vi "zad1.vi"() -> ()   [LabVIEW 2018]
uses:
  <vilib>/sound2/lvsound2.llb/Sampling Mode.ctl
  <vilib>/sound2/lvsound2.llb/Sound Data Format.ctl
  <vilib>/sound2/lvsound2.llb/Sound Output Set Volume (Single).vi
  <vilib>/sound2/lvsound2.llb/Sound Output Write (DBL Single).vi
  <vilib>/sound2/lvsound2.llb/Sound Input Read (DBL).vi
  <vilib>/measure/NI_MABase.lvlib
panel:
  in  "Stop":bool
  out "Waveform Graph 2":waveform(dbl)[](graph)
  out "Waveform Graph":waveform(dbl)(graph)
  in  "frequency":dbl(slide)=10.0 scale=200.0..2000.0
  in  "volume":dbl(knob)=100.0 scale=0.0..100.0
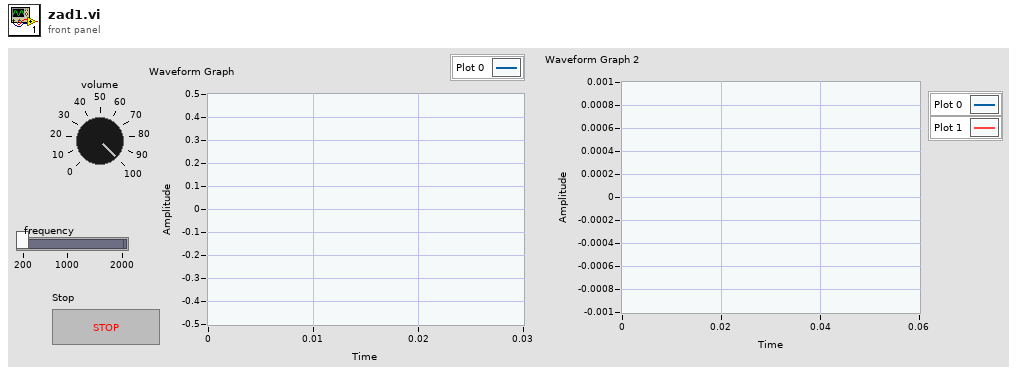
[diagram p1: front panel]
types:
  T1 = typedef "Sound Data Format.ctl" = cluster{"sample rate (S/s)":dbl, "number of channels":i32, "bits per sample":i32}
  T2 = typedef "Sampling Mode.ctl" = i32
  T3 = typedef "Sound Output Task ID.ctl" = u32
  T4 = typedef "Sound Input Task ID.ctl" = u32
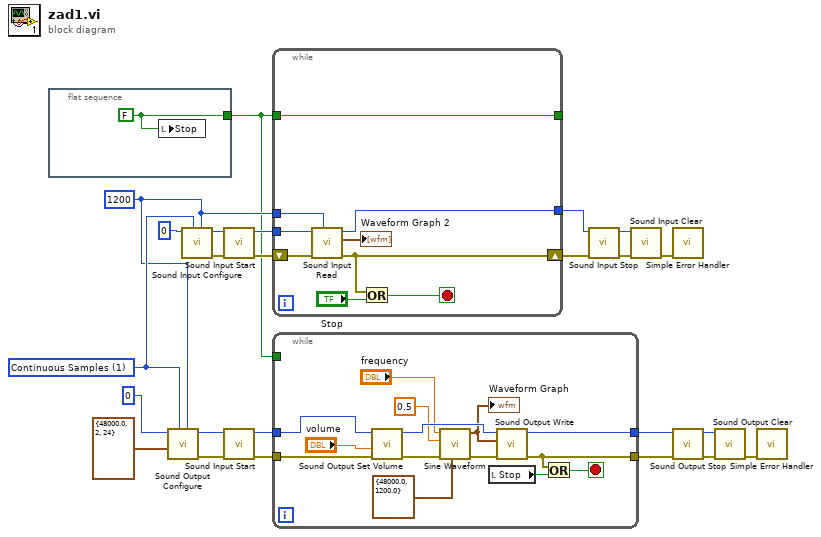
[diagram p0: block diagram]
diagram:
  w11 = 1200 ("number of samples/ch")
  w15 = T2 1 items=["Finite Samples", "Continuous Samples"] ("sample mode")
  n1 = flat-sequence {
    tunnel: [w25] -> w3
    frame #0 {
      w25 = FALSE
      n2 = local write "Stop"(w25) -> ()
    }
  }
  n3 = call <vilib>:"Sound Output Configure.vi"("number of samples/ch"=w11, "sample mode"=w15, "sound format"=T1 {"sample rate (S/s)"=48000.0, "number of channels"=2, "bits per sample"=24}, "device ID"=u32 0) -> ("error out"=w5:errorcluster, "task ID"=w6:T3)  [unwired: 6 in]
  n4 = call <vilib>:"Sound Input Configure.vi"("number of samples/ch"=w11, "sample mode"=w15, "device ID"=u32 0) -> ("error out"=w18:errorcluster, "task ID"=w19:T4)  [unwired: 7 in]
  n5 = call <vilib>:"Sound Input Start.vi"("error in (no error)"=w18, "task ID"=w19) -> ("error out"=w16:errorcluster, "task ID out"=w17:T4)  [unwired: 8 in]
  n6 = call <vilib>:"Sound Input Start.vi"("error in (no error)"=w5, "task ID"=w6) -> ("error out"=w7:errorcluster, "task ID out"=w8:T4)  [unwired: 8 in]
  n7 = while {
    tunnel: w17 -> [w34]
    tunnel: w11 -> [w31]
    shift-right: [w29] -> w10
    shift-left: w16 -> [w33]
    tunnel: [w27] -> w4
    tunnel: [w26] -> _
    tunnel: w3 -> [w26]
    stop <- w28 stop-if-true
    n8 = call-poly <vilib>:"Sound Input Read.vi"("number of samples/ch"=w31, "error in (no error)"=w33, "task ID"=w34) -> ("error out"=w29:errorcluster, "data"=→"Waveform Graph 2":waveform(dbl)[], "task ID out"=w27:T4)  [unwired: 6 in]
    n9 = Or(x=w29, y="Stop") -> (x .or. y?=w28:bool)
  }
  n10 = while {
    tunnel: w8 -> [w48]
    tunnel: w7 -> [w47]
    tunnel: [w38] -> w21
    tunnel: [w37] -> w20
    tunnel: w3 -> [_]
    stop <- w36 stop-if-true
    n11 = call-poly <vilib>:"Sound Output Set Volume.vi"("error in (no error)"=w47, "volume"="volume", "task ID"=w48) -> ("error out"=w44:errorcluster, "task ID out"=w45:T3)  [unwired: 7 in]
    n12 = call <vilib>:"Sine Waveform.vi"("sampling info"=cluster{"Fs":dbl, "#s":dbl} {"Fs"=48000.0, "#s"=1200.0}, "error in (no error)"=w44, "amplitude"=0.5 ("phase"), "frequency"="frequency") -> ("error out"=w43:errorcluster, "signal out"=w40:waveform(dbl))  [unwired: 6 in]
    "Waveform Graph" <- w40
    n13 = local read "Stop"() -> (w35:bool)
    n14 = call-poly <vilib>:"Sound Output Write.vi"("error in (no error)"=w43, "data"=w40, "task ID"=w45) -> ("error out"=w37:errorcluster, "task ID out"=w38:T3)  [unwired: 7 in]
    n15 = Or(x=w37, y=w35) -> (x .or. y?=w36:bool)
  }
  n16 = call <vilib>:"Sound Input Stop.vi"("error in (no error)"=w10, "task ID"=w4) -> ("error out"=w12:errorcluster, "task ID out"=w13:T4)  [unwired: 8 in]
  n17 = call <vilib>:"Sound Input Clear.vi"("error in (no error)"=w12, "task ID"=w13) -> ("error out"=w2:errorcluster)  [unwired: 9 in]
  n18 = call <vilib>:"Simple Error Handler.vi"("error in (no error)"=w2) -> ()  [unwired: 4 in, 5 out]
  n19 = call <vilib>:"Sound Output Stop.vi"("error in (no error)"=w20, "task ID"=w21) -> ("error out"=w23:errorcluster, "task ID out"=w22:T3)  [unwired: 8 in]
  n20 = call <vilib>:"Sound Output Clear.vi"("error in (no error)"=w23, "task ID"=w22) -> ("error out"=w1:errorcluster)  [unwired: 9 in]
  n21 = call <vilib>:"Simple Error Handler.vi"("error in (no error)"=w1) -> ()  [unwired: 4 in, 5 out]
